vi "Comm visa.vi"(8 "error in (no error)":errorcluster, 10 "Command":u8[](array[numeric]), 11 "VISA in":refnum<visa-resource-name>="COM7") -> (0 "error out":errorcluster, 1 "status log":string, 2 "Response":u8 format="%x", 3 "VISA out":refnum<visa-resource-name>)   [LabVIEW 2014, in "AISAS motor.lvclass"]
uses:
  AISAS motor.lvclass
  <vilib>/Instr/_visa.llb/VISA Flush IO Buffer Mask.ctl
panel:
  out "Response str":string
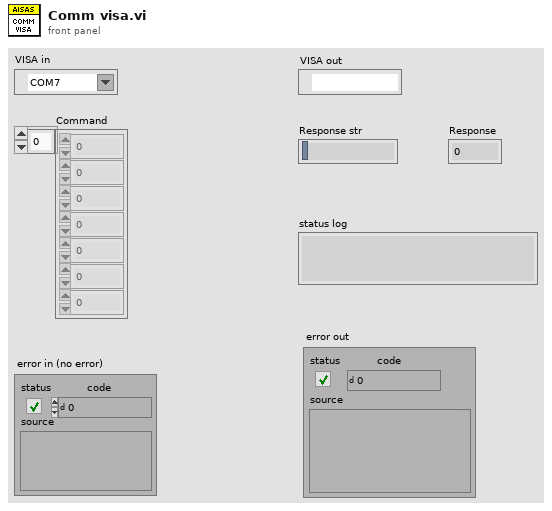
[diagram p1: front panel]
types:
  T1 = typedef "VISA Flush IO Buffer Mask.ctl" = u16
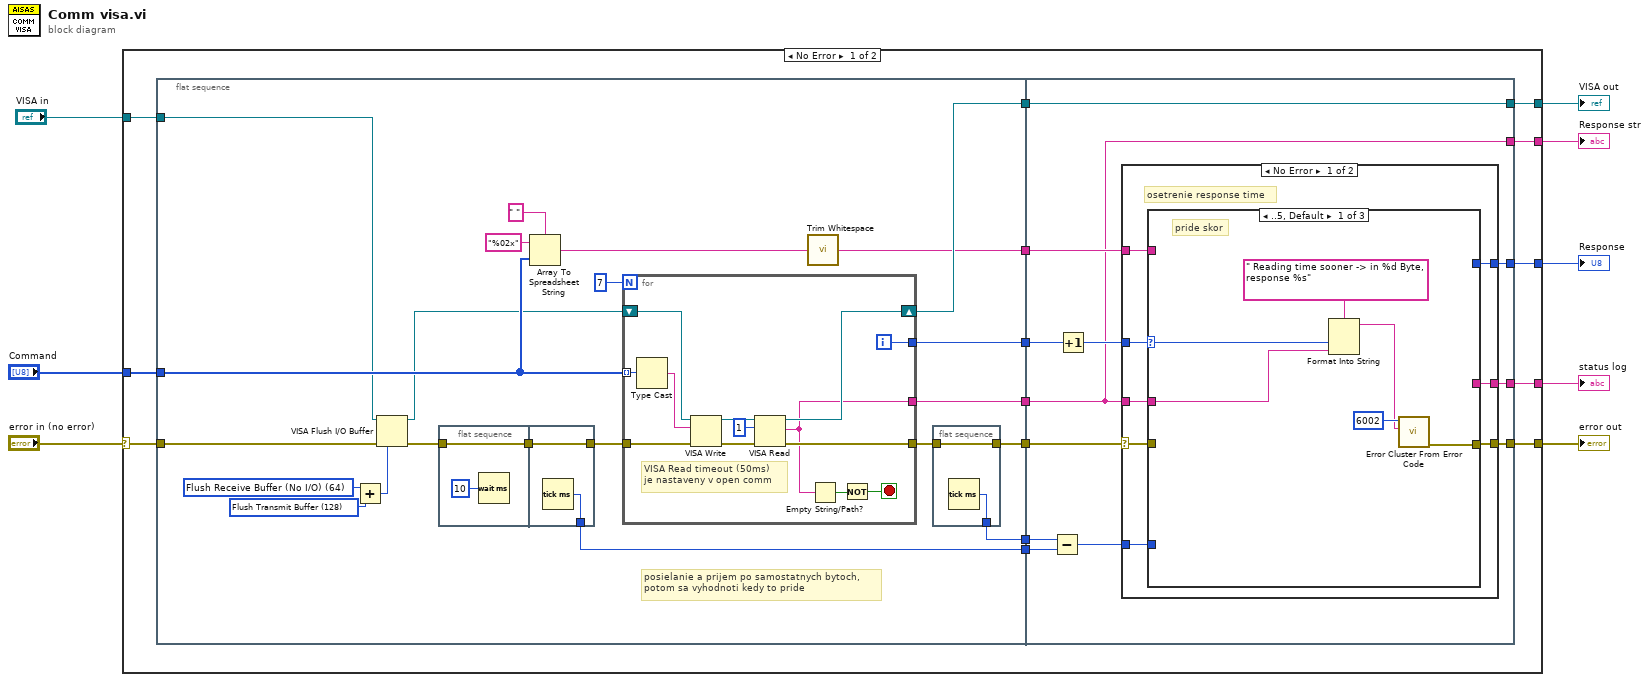
[diagram p0: block diagram]
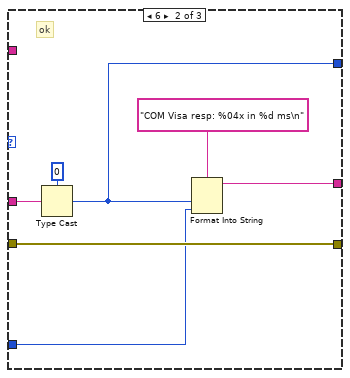
[diagram p2: hidden frame]
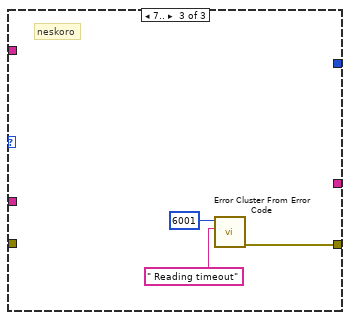
[diagram p3: hidden frame]
diagram:
  n1 = case shown="No Error" "error in (no error)" {
    selector: "error in (no error)" -> [w16 w103]
    tunnel: [w20 w103] -> w7
    tunnel: "Command" -> [w14 _]
    tunnel: "VISA in" -> [w13 w102]
    tunnel: [w12 _] -> w4
    tunnel: [w11 _] -> w3
    tunnel: [w10 w102] -> w2
    tunnel: [w9 _] -> w1
    frame No Error {
      n2 = flat-sequence {
        tunnel: [w45] -> w23
        tunnel: [w40] -> w22
        tunnel: [w43] -> w21
        tunnel: [w42] -> w19
        tunnel: [w39] -> w18
        tunnel: [w38] -> w17
        tunnel: w16 -> [w28]
        tunnel: [w33] -> w15
        tunnel: w14 -> [w32]
        tunnel: w13 -> [w26]
        tunnel: [w76] -> w20
        tunnel: w23 -> [w66]
        tunnel: w22 -> [w69]
        tunnel: w21 -> [w67]
        tunnel: w19 -> [w71]
        tunnel: w18 -> [w74]
        tunnel: w17 -> [w75]
        tunnel: w15 -> [w72]
        tunnel: [w68] -> w12
        tunnel: [w67] -> w11
        tunnel: [w66] -> w10
        tunnel: [w65] -> w9
        frame #0 {
          w30 = T1 128 items=["Flush Receive Buffer"=16, "Write Transmit Buffer to Device"=32, "Flush Receive Buffer (No I/O)"=64, "Flush Transmit Buffer"=128] ("y")
          w31 = T1 64 items=["Flush Receive Buffer"=16, "Write Transmit Buffer to Device"=32, "Flush Receive Buffer (No I/O)"=64, "Flush Transmit Buffer"=128] ("Mask")
          # "posielanie a prijem po samostatnych bytoch,\npotom sa vyhodnoti kedy to pride"
          n3 = Add(x=w31, y=w30) -> (x+y=w29:T1)
          n4 = VISA Flush I/O Buffer(VISA resource name=w26, mask (16)=w29, error in (no error)=w28) -> (VISA resource name out=w27:refnum<visa-resource-name>, error out=w25:errorcluster)
          n5 = flat-sequence {
            tunnel: w25 -> [w49]
            tunnel: [w49] -> w24
            tunnel: [w51] -> w39
            tunnel: [w50] -> w37
            tunnel: w24 -> [w50]
            frame #0 {
              n6 = Wait (ms)(milliseconds to wait=u32 10) -> ()  [unwired: 1 out]
            }
            frame #1 {
              n7 = Tick Count (ms)() -> (millisecond timer value=w51:u32)
            }
          }
          n8 = Array To Spreadsheet String(delimiter (Tab)=" ", array=w32, 3:"%02x" ("format string")) -> (spreadsheet string=w34:string)
          n9 = for {
            N: 7 -> [_]
            shift-right: [w64] -> w45
            shift-left: w27 -> [w63]
            tunnel: [w56] -> w43
            tunnel: [w61] -> w42
            tunnel: [w62] -> w41
            tunnel: w37 -> [w54]
            tunnel: w32 -> [w52] mode=indexing
            i -> [w61]
            stop <- w55 stop-if-true
            # "VISA Read timeout (50ms)\nje nastaveny v open comm"
            n10 = Type Cast(x=w52) -> (*(type *) &x=w53:string)  [unwired: 1 in]
            n11 = VISA Write(VISA resource name=w63, write buffer=w53, error in (no error)=w54) -> (VISA resource name out=w60:refnum<visa-resource-name>, error out=w59:errorcluster)  [unwired: 1 out]
            n12 = VISA Read(VISA resource name=w60, byte count=u32 1, error in (no error)=w59) -> (VISA resource name out=w64:refnum<visa-resource-name>, read buffer=w56:string, error out=w62:errorcluster)  [unwired: 1 out]
            n13 = Empty String/Path?(string/path=w56) -> (empty?=w57:bool)
            n14 = Not(x=w57) -> (.not. x?=w55:bool)
          }
          n15 = call <vilib>:"Trim Whitespace.vi"("string"=w34) -> ("trimmed string"=w33:string)  [unwired: 1 in]
          n16 = flat-sequence {
            tunnel: w41 -> [w47]
            tunnel: [w47] -> w40
            tunnel: [w46] -> w38
            frame #0 {
              n17 = Tick Count (ms)() -> (millisecond timer value=w46:u32)
            }
          }
        }
        frame #1 {
          n18 = Subtract(x=w75, y=w74) -> (x-y=w73:u32)
          n19 = Increment(x=w71) -> (x+1=w70:i32)
          n20 = case shown="No Error" w69 {
            selector: w69 -> [w79 w101]
            tunnel: w67 -> [w84 _]
            tunnel: [w83 w101] -> w76
            tunnel: w73 -> [w82 _]
            tunnel: w72 -> [w81 _]
            tunnel: w70 -> [w80 _]
            tunnel: [w78 _] -> w68
            tunnel: [w77 _] -> w65
            frame No Error {
              # "osetrenie response time"
              n21 = case shown="..5, Default" w80 {
                selector: w80 -> [w87 _ _]
                tunnel: w79 -> [_ w97 _]
                tunnel: [w89 w97 w98] -> w83
                tunnel: w84 -> [w85 w94 _]
                tunnel: w82 -> [_ w93 _]
                tunnel: w81 -> [_ _ _]
                tunnel: [_ w92 _] -> w78
                tunnel: [_ w91 _] -> w77
                frame ..5, Default {
                  # "pride skor"
                  n22 = Format Into String(format string=" Reading time sooner -> in %d Byte, response %s" ("error message (\"\")"), w87, w85) -> (resulting string=w86:string)  [unwired: 2 in, 1 out]
                  n23 = call <vilib>:"Error Cluster From Error Code.vi"("error message (\"\")"=w86, "error code (0)"=6002) -> ("error out"=w89:errorcluster)  [unwired: 7 in]
                }
                frame 6 {
                  # "ok"
                  n24 = Type Cast(type=u8 0, x=w94) -> (*(type *) &x=w91:u8)
                  n25 = Format Into String(format string="COM Visa resp: %04x in %d ms\n" ("read buffer"), w91, w93) -> (resulting string=w92:string)  [unwired: 2 in, 1 out]
                }
                frame 7.. {
                  # "neskoro"
                  n26 = call <vilib>:"Error Cluster From Error Code.vi"("error message (\"\")"=" Reading timeout" ("error message (\"\")"), "error code (0)"=6001) -> ("error out"=w98:errorcluster)  [unwired: 7 in]
                }
              }
            }
            frame Error {
            }
          }
        }
      }
    }
    frame Error {
    }
  }
  "error out" <- w7
  "status log" <- w4
  "Response str" <- w3
  "VISA out" <- w2
  "Response" <- w1
